vi "Escribir_Dato_Excel.vi"   [LabVIEW 2020]
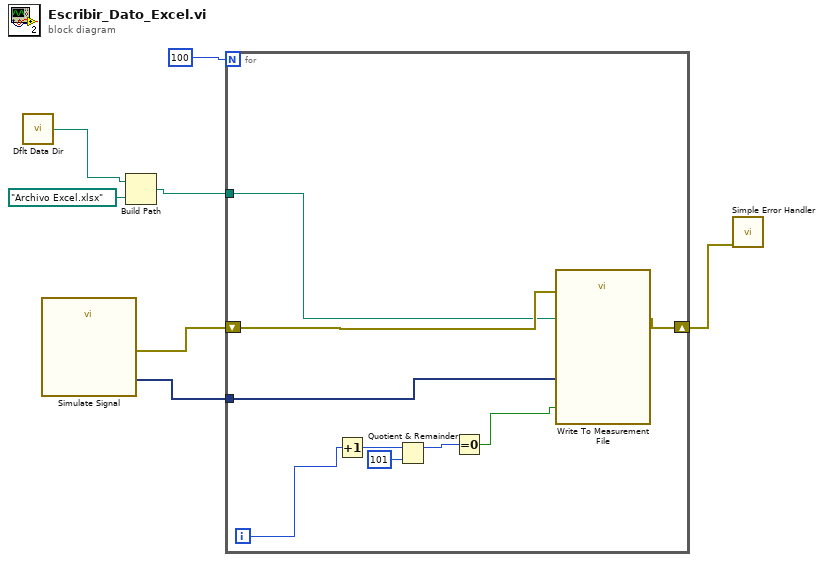
[diagram p0: block diagram]
diagram:
  n1 = call <vilib>:"Dflt Data Dir.vi"() -> ("App:Default Data Directory"=w1:path)
  n2 = call "Simulate Signal"() -> ("Sine"=w7:dynamicdata, "error out"=w5:errorcluster)  [unwired: 14 in]
  n3 = Build Path(base path=w1, name or relative path=path "Archivo Excel.xlsx") -> (appended path=w3:path)
  n4 = for {
    N: 100 -> [_]
    tunnel: w7 -> [w16]
    shift-right: [w14] -> w4
    shift-left: w5 -> [w15]
    tunnel: w3 -> [w13]
    i -> [w9]
    n5 = Increment(x=w9) -> (x+1=w12:i32)
    n6 = Quotient & Remainder(x=w12, y=101) -> (x-y*floor(x/y)=w11:i32)  [unwired: 1 out]
    n7 = Equal To 0?(x=w11) -> (x = 0?=w8:bool)
    n8 = call "Write To Measurement File"("Signals"=w16, "Flush? (T)"=w8, "error in (no error)"=w15, "Filename"=w13) -> ("error out"=w14:errorcluster)  [unwired: 13 in, 2 out]
  }
  n9 = call <vilib>:"Simple Error Handler.vi"("error in (no error)"=w4) -> ()  [unwired: 4 in, 5 out]
